vi "Execute.vi"(8 "error in (no error)":errorcluster, 10 "Abstract Consumer in":refnum<class "Abstract Consumer.lvclass">, 11 "Switch Disconnect Message in":refnum<class "Switch Disconnect Message.lvclass">) -> (0 "error out":errorcluster, 1 "Abstract Response out":refnum<class "Abstract Response Message.lvclass">, 2 "Abstract Consumer out":refnum<class "Abstract Consumer.lvclass">, 3 "Switch Disconnect Message out":refnum<class "Switch Disconnect Message.lvclass">, 4 "Stop?":bool)   [LabVIEW 2017, in "Messaging.lvlib" / "Switch Disconnect Message.lvclass"]
uses:
  Switch Disconnect Message.lvclass
  Consumer/Abstract Consumer/Abstract Consumer.lvclass
  Message/Abstract Response Message/Abstract Response Message.lvclass
  Abstract Switch Consumer/Abstract Switch Consumer.lvclass
  C:/github/niveristand-custom-device-message-library/Source/Consumer/Abstract Consumer/Abstract Consumer.lvclass
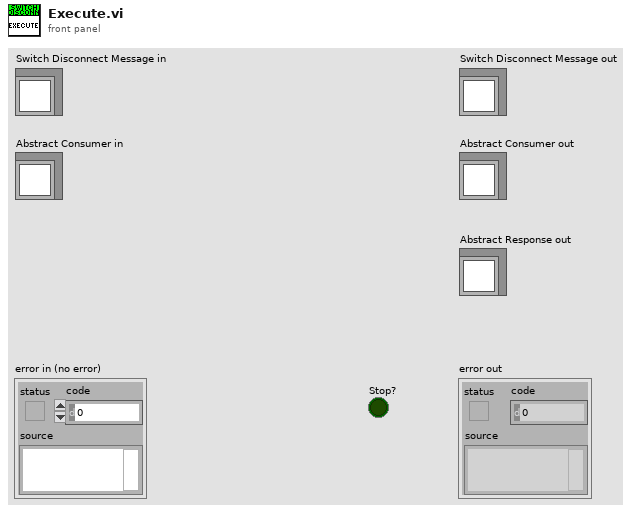
[diagram p1: front panel]
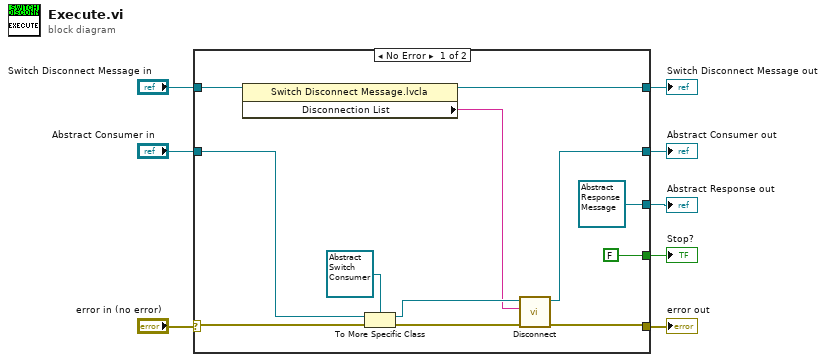
[diagram p0: block diagram]
diagram:
  n1 = case shown="No Error" "error in (no error)" {
    selector: "error in (no error)" -> [w14 w23]
    tunnel: [w13 w23] -> w7
    tunnel: [w10 w22] -> w6
    tunnel: "Switch Disconnect Message in" -> [w16 w22]
    tunnel: [w11 w21] -> w4
    tunnel: "Abstract Consumer in" -> [w15 w21]
    tunnel: [FALSE ("Stop?") _] -> w2
    tunnel: [refnum<class "Abstract Response Message.lvclass"> refnum ("Abstract Response out") _] -> w1
    frame No Error {
      n2 = property class="Switch Disconnect Message.lvcla"(reference=w16) -> (reference out=w10:refnum<class "Switch Disconnect Message.lvclass">, "Disconnection List"=w17:string)  [unwired: 1 in, 1 out]
      n3 = To More Specific Class(target class=refnum<class "Abstract Switch Consumer.lvclass"> refnum ("Message Queue Library.lvlib:Abstract Switch Consumer.lvclass"), reference=w15, error in=w14) -> (specific class reference=w18:refnum<class "Abstract Switch Consumer.lvclass">, error out=w19:errorcluster)
      n4 = call-dynamic "Disconnect.vi"("error in (no error)"=w19, "Disconnection list in"=w17, "Abstract Switch Consumer in"=w18) -> ("error out"=w13:errorcluster, "Abstract Switch Consumer out"=w11:refnum<class "Abstract Switch Consumer.lvclass">)  [unwired: 7 in]
    }
    frame Error {
    }
  }
  "error out" <- w7
  "Switch Disconnect Message out" <- w6
  "Abstract Consumer out" <- w4
  "Stop?" <- w2
  "Abstract Response out" <- w1
